vi "Finish.vi"   [LabVIEW 2018]
doc: "This VI is called just before exiting. It is expected to close I/O refnum, save collected data, etc."
uses:
  <vilib>/Rock Robotics/WPI/Utilities/WPI_GetSetVariantRefNum.vi
types:
  T1 = typedef "WPI_JoystickDevRef.ctl" = cluster{"Device":T2}
  T2 = typedef "WPI_JoystickDeviceEnum.ctl" = enum16{"USB 0", "USB 1", "USB 2", "USB 3", "USB 4", "USB 5"}
  T3 = typedef "WPI_CompressorDevRef.ctl" = cluster{"DevStatus":errorcluster, "Pneumatics Control Module":u8}
  T4 = typedef "WPI_SolenoidDevRef.ctl" = cluster{"DevStatus":errorcluster, "Pneumatics Control Module":u8, "Forward Solenoid Channel":T5, "Reverse Solenoid Channel":T5}
  T5 = typedef "WPI_SolenoidChannel.ctl" = enum8{"Solenoid 0", "Solenoid 1", "Solenoid 2", "Solenoid 3", "Solenoid 4", "Solenoid 5", "Solenoid 6", "Solenoid 7", "Invalid"}
  T6 = typedef "WPI_MotorControlDeviceRef.ctl" = cluster{"DeviceStatus":errorcluster, "Type":T7, "PWM":cluster{"PWM Channel":T8, "DeadBand":T9}, "CAN":cluster{"Device Number":u8, "SetOutput VI Ref":variant, "GetOutput VI Ref":variant, "Enable VI Ref":variant, "Disable VI Ref":variant, "Data":variant}, "Invert":bool, "DIO PWM":cluster{"PWM \"Enable\" Channel":T8, "DIOChannel":T10, "PWM Rate":dbl}}
  T7 = typedef "WPI_MotorControlType.ctl" = enum16{"PWM", "CAN", "DIO PWM"}
  T8 = typedef "FPGA_DIOPWMChannel.ctl" = enum8{"PWM 0", "PWM 1", "PWM 2", "PWM 3", "PWM 4", "PWM 5", "PWM 6", "PWM 7", "PWM 8", "PWM 9", "PWM MXP 0", "PWM MXP 1", "PWM MXP 2", "PWM MXP 3", "PWM MXP 4", "PWM MXP 5", "PWM MXP 6", "PWM MXP 7", "PWM MXP 8", "PWM MXP 9", "Invalid"}
  T9 = typedef "WPI_PWMDeadband.ctl" = cluster{"Name":string, "maxPositivePwm":i32, "minPositivePwm":i32, "centerPwm":i32, "maxNegativePwm":i32, "minNegativePwm":i32, "angularRange":u16}
  T10 = typedef "FPGA_DIOChannel.ctl" = enum8{"DIO 0", "DIO 1", "DIO 2", "DIO 3", "DIO 4", "DIO 5", "DIO 6", "DIO 7", "DIO 8", "DIO 9", "DIO MXP 0", "DIO MXP 1", "DIO MXP 2", "DIO MXP 3", "DIO MXP 4", "DIO MXP 5", "DIO MXP 6", "DIO MXP 7", "DIO MXP 8", "DIO MXP 9", "DIO MXP 10", "DIO MXP 11", "DIO MXP 12", "DIO MXP 13", "DIO MXP 14", "DIO MXP 15", "SPI Port CS1", "SPI Port CS2", "SPI Port CS3", "SPI Port MISO", "SPI Port MOSI", "Invalid"}
  T11 = typedef "WPI_RobotDriveDevRef.ctl" = cluster{"DevStatus":errorcluster, "Motors[]":T6[], "Square Inputs":bool, "Max Output":dbl}
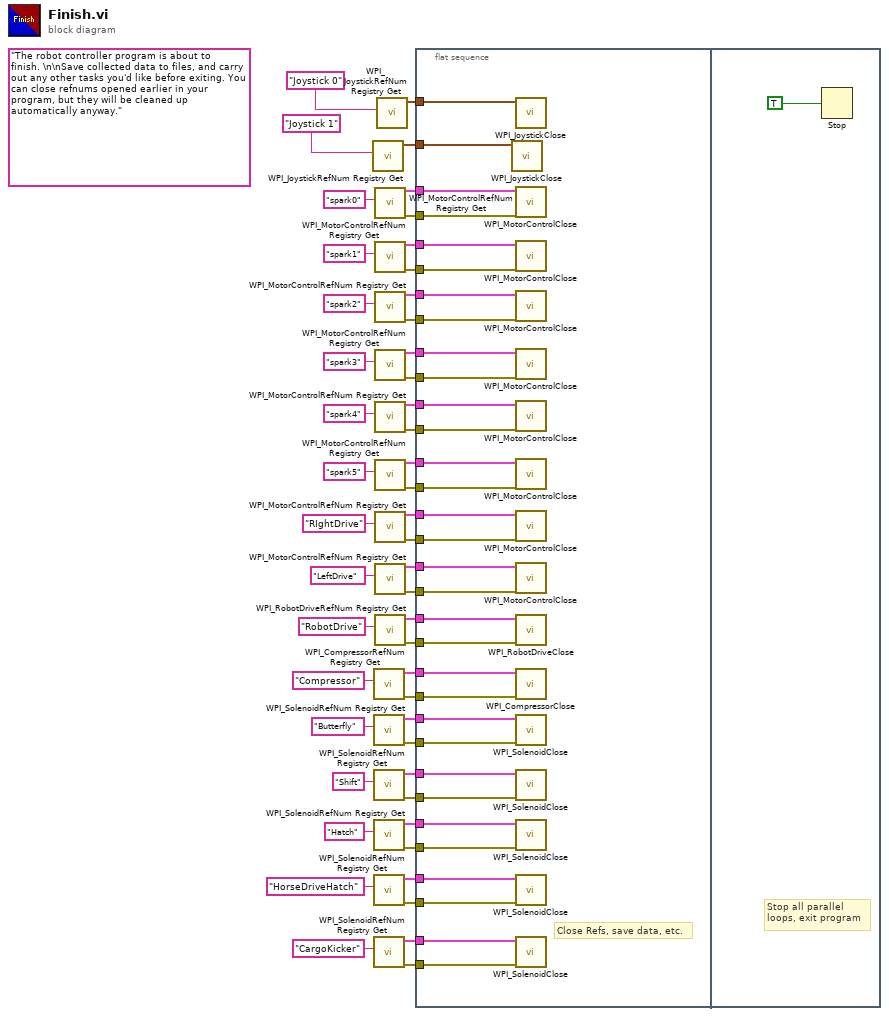
[diagram p0: block diagram]
diagram:
  (unwired) "The robot controller program is about to finish. \n\nSave collected data to files, and carry out any other tasks you'd like before exiting. You can close refnums opened earlier in your program, but they will be cleaned up automatically anyway."
  n1 = call <vilib>:"WPI_JoystickRefNum Registry Get.vi"("refnum name"="Joystick 1") -> ("JoystickDevRef"=w2:T1)  [unwired: 1 in, 9 out]
  n2 = call <vilib>:"WPI_CompressorRefNum Registry Get.vi"("refnum name"="Compressor") -> ("error out"=w18:errorcluster, "CompressorDevRef"=w19:T3)  [unwired: 9 in]
  n3 = call <vilib>:"WPI_SolenoidRefNum Registry Get.vi"("refnum name"="Butterfly") -> ("error out"=w16:errorcluster, "SolenoidDevRef"=w17:T4)  [unwired: 9 in]
  n4 = call <vilib>:"WPI_SolenoidRefNum Registry Get.vi"("refnum name"="Shift") -> ("error out"=w13:errorcluster, "SolenoidDevRef"=w12:T4)  [unwired: 9 in]
  n5 = call <vilib>:"WPI_SolenoidRefNum Registry Get.vi"("refnum name"="Hatch") -> ("error out"=w7:errorcluster, "SolenoidDevRef"=w6:T4)  [unwired: 9 in]
  n6 = call <vilib>:"WPI_SolenoidRefNum Registry Get.vi"("refnum name"="HorseDriveHatch") -> ("error out"=w10:errorcluster, "SolenoidDevRef"=w11:T4)  [unwired: 9 in]
  n7 = call <vilib>:"WPI_SolenoidRefNum Registry Get.vi"("refnum name"="CargoKicker") -> ("error out"=w4:errorcluster, "SolenoidDevRef"=w3:T4)  [unwired: 9 in]
  n8 = call <vilib>:"WPI_MotorControlRefNum Registry Get.vi"("refnum name"="spark0") -> ("error out"=w46:errorcluster, "MotorControlDevRef"=w47:T6)  [unwired: 9 in]
  n9 = call <vilib>:"WPI_MotorControlRefNum Registry Get.vi"("refnum name"="spark1") -> ("error out"=w43:errorcluster, "MotorControlDevRef"=w42:T6)  [unwired: 9 in]
  n10 = call <vilib>:"WPI_MotorControlRefNum Registry Get.vi"("refnum name"="spark2") -> ("error out"=w40:errorcluster, "MotorControlDevRef"=w41:T6)  [unwired: 9 in]
  n11 = call <vilib>:"WPI_MotorControlRefNum Registry Get.vi"("refnum name"="spark3") -> ("error out"=w37:errorcluster, "MotorControlDevRef"=w36:T6)  [unwired: 9 in]
  n12 = call <vilib>:"WPI_MotorControlRefNum Registry Get.vi"("refnum name"="spark4") -> ("error out"=w34:errorcluster, "MotorControlDevRef"=w35:T6)  [unwired: 9 in]
  n13 = call <vilib>:"WPI_MotorControlRefNum Registry Get.vi"("refnum name"="spark5") -> ("error out"=w31:errorcluster, "MotorControlDevRef"=w30:T6)  [unwired: 9 in]
  n14 = call <vilib>:"WPI_MotorControlRefNum Registry Get.vi"("refnum name"="RIghtDrive") -> ("error out"=w25:errorcluster, "MotorControlDevRef"=w26:T6)  [unwired: 9 in]
  n15 = call <vilib>:"WPI_MotorControlRefNum Registry Get.vi"("refnum name"="LeftDrive") -> ("error out"=w28:errorcluster, "MotorControlDevRef"=w27:T6)  [unwired: 9 in]
  n16 = call <vilib>:"WPI_RobotDriveRefNum Registry Get.vi"("refnum name"="RobotDrive") -> ("error out"=w22:errorcluster, "RobotDriveDevRef"=w23:T11)  [unwired: 9 in]
  n17 = call <vilib>:"WPI_JoystickRefNum Registry Get.vi"("refnum name"="Joystick 0") -> ("JoystickDevRef"=w48:T1)  [unwired: 1 in, 9 out]
  n18 = flat-sequence {
    tunnel: w48 -> [w81]
    tunnel: w47 -> [w80]
    tunnel: w46 -> [w79]
    tunnel: w42 -> [w77]
    tunnel: w43 -> [w78]
    tunnel: w41 -> [w76]
    tunnel: w40 -> [w75]
    tunnel: w36 -> [w73]
    tunnel: w37 -> [w74]
    tunnel: w35 -> [w72]
    tunnel: w34 -> [w71]
    tunnel: w30 -> [w69]
    tunnel: w31 -> [w70]
    tunnel: w26 -> [w66]
    tunnel: w25 -> [w65]
    tunnel: w27 -> [w67]
    tunnel: w28 -> [w68]
    tunnel: w23 -> [w64]
    tunnel: w22 -> [w63]
    tunnel: w19 -> [w62]
    tunnel: w18 -> [w61]
    tunnel: w17 -> [w60]
    tunnel: w16 -> [w59]
    tunnel: w12 -> [w57]
    tunnel: w13 -> [w58]
    tunnel: w6 -> [w53]
    tunnel: w7 -> [w54]
    tunnel: w11 -> [w56]
    tunnel: w10 -> [w55]
    tunnel: w3 -> [w51]
    tunnel: w4 -> [w52]
    tunnel: w2 -> [w50]
    frame #0 {
      # "Close Refs, save data, etc."
      n19 = call <vilib>:"WPI_JoystickClose.vi"("JoystickDevRef"=w50) -> ()  [unwired: 11 out]
      n20 = call <vilib>:"WPI_JoystickClose.vi"("JoystickDevRef"=w81) -> ()  [unwired: 11 out]
      n21 = call <vilib>:"WPI_MotorControlClose.vi"("error in"=w79, "MotorControlDevRef"=w80) -> ()  [unwired: 9 in, 1 out]
      n22 = call <vilib>:"WPI_MotorControlClose.vi"("error in"=w78, "MotorControlDevRef"=w77) -> ()  [unwired: 9 in, 1 out]
      n23 = call <vilib>:"WPI_MotorControlClose.vi"("error in"=w75, "MotorControlDevRef"=w76) -> ()  [unwired: 9 in, 1 out]
      n24 = call <vilib>:"WPI_MotorControlClose.vi"("error in"=w74, "MotorControlDevRef"=w73) -> ()  [unwired: 9 in, 1 out]
      n25 = call <vilib>:"WPI_MotorControlClose.vi"("error in"=w71, "MotorControlDevRef"=w72) -> ()  [unwired: 9 in, 1 out]
      n26 = call <vilib>:"WPI_MotorControlClose.vi"("error in"=w70, "MotorControlDevRef"=w69) -> ()  [unwired: 9 in, 1 out]
      n27 = call <vilib>:"WPI_MotorControlClose.vi"("error in"=w65, "MotorControlDevRef"=w66) -> ()  [unwired: 9 in, 1 out]
      n28 = call <vilib>:"WPI_MotorControlClose.vi"("error in"=w68, "MotorControlDevRef"=w67) -> ()  [unwired: 9 in, 1 out]
      n29 = call <vilib>:"WPI_RobotDriveClose.vi"("error in (no error)"=w63, "RobotDriveDevRef"=w64) -> ()  [unwired: 9 in, 1 out]
      n30 = call <vilib>:"WPI_CompressorClose.vi"("error in (no error)"=w61, "CompressorDevRef"=w62) -> ()  [unwired: 9 in, 1 out]
      n31 = call <vilib>:"WPI_SolenoidClose.vi"("error in (no error)"=w59, "SolenoidDevRef"=w60) -> ()  [unwired: 9 in, 1 out]
      n32 = call <vilib>:"WPI_SolenoidClose.vi"("error in (no error)"=w58, "SolenoidDevRef"=w57) -> ()  [unwired: 9 in, 1 out]
      n33 = call <vilib>:"WPI_SolenoidClose.vi"("error in (no error)"=w54, "SolenoidDevRef"=w53) -> ()  [unwired: 9 in, 1 out]
      n34 = call <vilib>:"WPI_SolenoidClose.vi"("error in (no error)"=w55, "SolenoidDevRef"=w56) -> ()  [unwired: 9 in, 1 out]
      n35 = call <vilib>:"WPI_SolenoidClose.vi"("error in (no error)"=w52, "SolenoidDevRef"=w51) -> ()  [unwired: 9 in, 1 out]
    }
    frame #1 {
      # "Stop all parallel\nloops, exit program"
      n36 = Stop(stop? (T)=TRUE ("Quit")) -> ()
    }
  }
